vi "ExampleReader.vi"() -> ()   [LabVIEW 2013]
uses:
  Reader/readType.ctl
  HelperVIs/EStopAction.ctl
  Reader/NetworkStreamReader.lvclass
panel:
  out "Connected? 2":bool
  out "Connected?":bool
  out "Cluster":T1
  out "Iteration Time Stamp":timestamp
  out "OCU Time Stamp":timestamp
  in  "stop":bool
  in  "Read Type":T2=enum."Most current"
  in  "Loop delay (ms)":u32=10
  out "element":variant
  out "data":i32
  # "Note: writer is running at 50 ms"
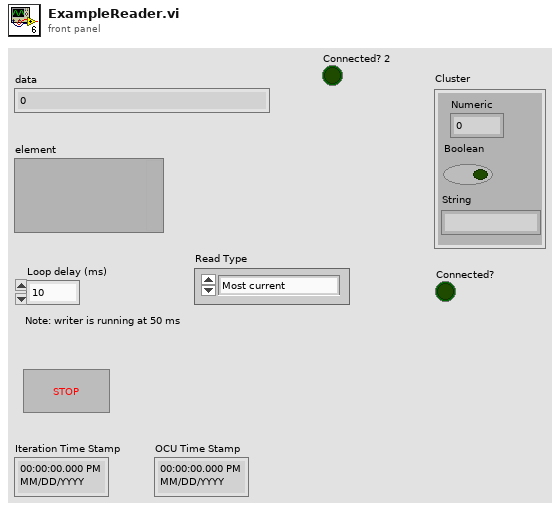
[diagram p1: front panel]
types:
  T1 = cluster{"Numeric":dbl, "Boolean":bool, "String":string}
  T2 = typedef "NetworkStreamReader.lvclass/readType.ctl" = enum16{"Next in buffer", "Most current"}
  T3 = typedef "EStopAction.ctl" = enum16{"Get", "Set"}
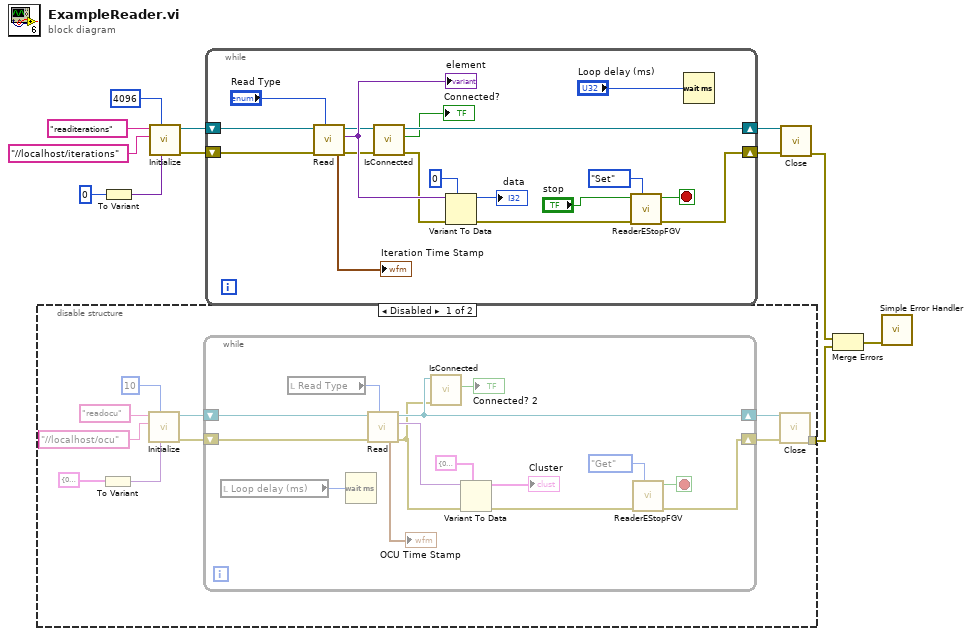
[diagram p0: block diagram]
diagram:
  n1 = disable-structure shown="Disabled" {
    disable-tunnel: [w16 _] -> w11
    frame Disabled {
      n2 = To Variant(anything=T1 {"Numeric"=0.0, "Boolean"=FALSE, "String"=""} ("Cluster")) -> (Variant=w22:variant)
      n3 = call "Initialize.vi"("Default return"=w22, "reader buffer size"=10 ("writer buffer size"), "writer url"="//localhost/ocu", "reader name"="readocu") -> ("error out"=w17:errorcluster, "NetworkStreamWriter out"=w19:refnum<class "NetworkStreamReader.lvclass">)  [unwired: 6 in]
      n4 = while {
        shift-right: [w26] -> w21
        shift-left: w19 -> [w37]
        shift-right: [w27] -> w20
        shift-left: w17 -> [w36]
        stop <- w23 stop-if-true
        n5 = local read "Loop delay (ms)"() -> (w33:u32)
        n6 = local read "Read Type"() -> (w34:T2)
        n7 = Wait (ms)(milliseconds to wait=w33) -> ()  [unwired: 1 out]
        n8 = call "Read.vi"("Read Type"=w34, "error in (no error)"=w36, "NetworkStreamReader in"=w37) -> ("error out"=w25:errorcluster, "element"=w35:variant, "NetworkStreamReader out"=w26:refnum<class "NetworkStreamReader.lvclass">, "Time Stamp"=→"OCU Time Stamp":timestamp)  [unwired: 4 in, 1 out]
        n9 = call "IsConnected.vi"("error in (no error)"=w25, "NetworkStreamReader in"=w26) -> ("Connected?"=→"Connected? 2":bool)  [unwired: 7 in, 2 out]
        n10 = Variant To Data(error in=w25, type=T1 {"Numeric"=0.0, "Boolean"=FALSE, "String"=""} ("Cluster"), Variant=w35) -> (data=→"Cluster":T1, error out=w28:errorcluster)
        n11 = call "ReaderEStopFGV.vi"("E-Stop Action"=EStopAction."Get", "Error In"=w28) -> ("Error Out"=w27:errorcluster, "E-Stop Out"=w23:bool)  [unwired: 8 in]
      }
      n12 = call "Close.vi"("error in (no error)"=w20, "NetworkStreamReader in"=w21) -> ("error out"=w16:errorcluster)  [unwired: 9 in]
    }
    frame Enabled {
    }
  }
  n13 = To Variant(anything=0) -> (Variant=w3:variant)
  n14 = call "Initialize.vi"("Default return"=w3, "reader buffer size"=4096 ("writer buffer size"), "writer url"="//localhost/iterations", "reader name"="readiterations") -> ("error out"=w9:errorcluster, "NetworkStreamWriter out"=w7:refnum<class "NetworkStreamReader.lvclass">)  [unwired: 6 in]
  n15 = while {
    shift-right: [w40] -> w5
    shift-left: w7 -> [w55]
    shift-right: [w44] -> w6
    shift-left: w9 -> [w54]
    stop <- w45 stop-if-true
    n16 = call "Read.vi"("Read Type"="Read Type", "error in (no error)"=w54, "NetworkStreamReader in"=w55) -> ("error out"=w42:errorcluster, "element"=w53:variant, "NetworkStreamReader out"=w43:refnum<class "NetworkStreamReader.lvclass">, "Time Stamp"=→"Iteration Time Stamp":timestamp)  [unwired: 4 in, 1 out]
    "element" <- w53
    n17 = call "IsConnected.vi"("error in (no error)"=w42, "NetworkStreamReader in"=w43) -> ("error out"=w41:errorcluster, "Connected?"=→"Connected?":bool, "NetworkStreamReader out"=w40:refnum<class "NetworkStreamReader.lvclass">)  [unwired: 7 in]
    n18 = Variant To Data(error in=w41, type=0, Variant=w53) -> (data=→"data":i32, error out=w46:errorcluster)
    n19 = call "ReaderEStopFGV.vi"("E-Stop Action"=EStopAction."Set", "Error In"=w46, "E-Stop In"="stop") -> ("Error Out"=w44:errorcluster, "E-Stop Out"=w45:bool)  [unwired: 7 in]
    n20 = Wait (ms)(milliseconds to wait="Loop delay (ms)") -> ()  [unwired: 1 out]
  }
  n21 = call "Close.vi"("error in (no error)"=w6, "NetworkStreamReader in"=w5) -> ("error out"=w12:errorcluster)  [unwired: 9 in]
  n22 = Merge Errors(w12, w11) -> (w10:errorcluster)
  n23 = call <vilib>:"Simple Error Handler.vi"("error in (no error)"=w10) -> ()  [unwired: 4 in, 5 out]
